vi "Load From XML.vi"(8 "error in":errorcluster, 10 "XML file path":path, 11 "state in":T1) -> (0 "error out":errorcluster, 1 "loaded?":bool, 2 "layout keyword":string, 3 "state out":T1)   [LabVIEW 2010, in "NI_SE_Config Front Panel Layout.lvlib"]
uses:
  NI_SE_Config Front Panel Layout.lvlib
  State.ctl
  VI Info.ctl
  VI Panel Layout/VI Panel Layout.lvclass
  VI Panel Layout/VI Panel Layout.lvclass/VI Panel Layout.ctl
  VI Panel Layout/Get Subpanel VIs.vi
  Check File Path.vi
  XML File Path to VI File Path.vi
  File Name to Width_Height.vi
  <vilib>/Utility/libraryn.llb/Check if File or Folder Exists.vi
  NI_SE_Front Panel Layout.lvlib
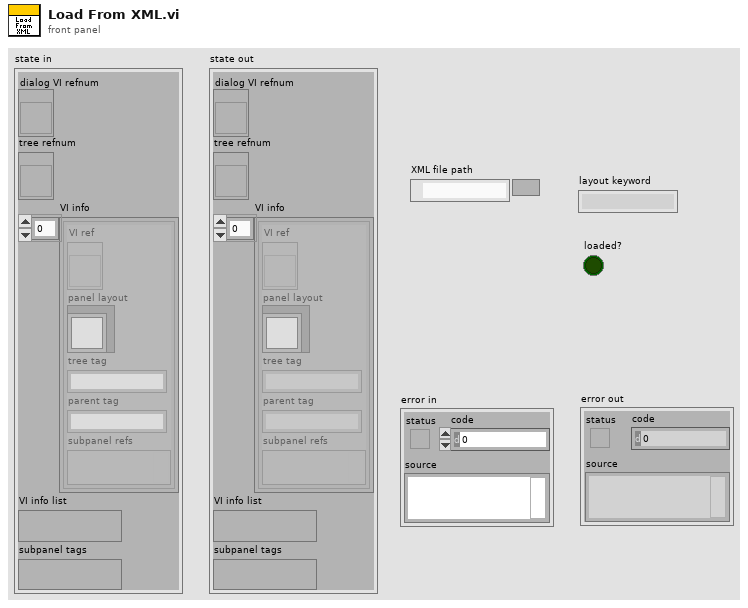
[diagram p1: front panel]
types:
  T1 = typedef "NI_SE_Config Front Panel Layout.lvlib/State.ctl" = cluster{"dialog VI refnum":refnum<vi>, "tree refnum":refnum<vi>, "VI info":T2[], "VI info list":variant, "subpanel tags":variant}
  T2 = typedef "NI_SE_Config Front Panel Layout.lvlib/VI Info.ctl" = cluster{"VI ref":refnum<vi>, "panel layout":refnum<class "VI Panel Layout.lvclass">, "tree tag":string, "parent tag":string, "subpanel refs":variant}
  T3 = typedef "LVBoundsTypeDef.ctl" = cluster{"Width":u32, "Height":u32}
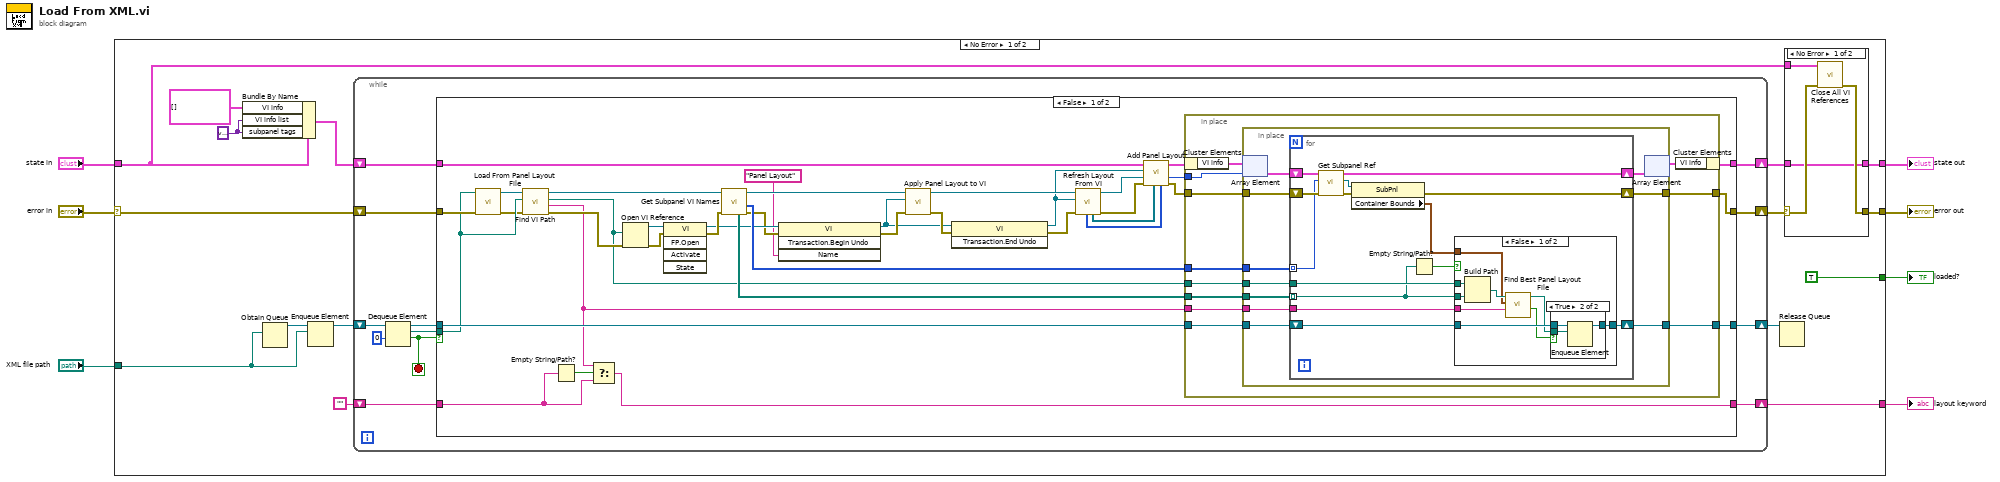
[diagram p0: block diagram]
diagram:
  n1 = case shown="No Error" "error in" {
    selector: "error in" -> [w23 w133]
    tunnel: "state in" -> [w16 w134]
    tunnel: [w8 w134] -> w5
    tunnel: [w14 w133] -> w4
    tunnel: "XML file path" -> [w21 _]
    tunnel: [w12 _] -> w2
    tunnel: [TRUE _] -> w1
    frame No Error {
      w18 = variant ("VI info list")
      n2 = Bundle By Name(cluster=w16, "VI info"=T2[] [], "VI info list"=w18, "subpanel tags"=w18) -> (w15:T1)
      n3 = Obtain Queue(element data type=w21) -> (queue out=w22:refnum<queue>)  [unwired: 4 in, 2 out]
      n4 = Enqueue Element(queue=w22, element=w21) -> (queue out=w20:refnum<queue>)  [unwired: 2 in, 2 out]
      n5 = while {
        shift-right: [w36] -> w19
        shift-left: w20 -> [w40]
        shift-right: [w33] -> w9
        shift-left: w15 -> [w34]
        shift-right: [w32] -> w10
        shift-left: w23 -> [w41]
        shift-right: [w30] -> w12
        shift-left: "" -> [w31]
        stop <- w35 stop-if-true
        n6 = Dequeue Element(queue=w40, timeout in ms (-1)=0) -> (queue out=w37:refnum<queue>, element=w38:path, timed out?=w35:bool)  [unwired: 1 in, 1 out]
        n7 = case shown="False" w35 {
          tunnel: w41 -> [w58 w130]
          tunnel: w38 -> [w54 _]
          tunnel: w37 -> [w78 w132]
          tunnel: [w77 w132] -> w36
          tunnel: w34 -> [w67 w131]
          tunnel: [w65 w131] -> w33
          tunnel: [w61 w130] -> w32
          tunnel: w31 -> [w73 w129]
          tunnel: [w74 w129] -> w30
          frame False {
            n8 = call "Load From Panel Layout File.vi"("error in"=w58, "panel layout file"=w54) -> ("error out"=w53:errorcluster, "panel layout out"=w56:refnum<class "VI Panel Layout.lvclass">)  [unwired: 8 in]
            n9 = call "Find VI Path.vi"("error in (no error)"=w53, "XML path (absolute)"=w54, "VI Panel Layout in"=w56) -> ("error out"=w52:errorcluster, "keyword"=w50:string, "VI path (absolute)"=w51:path, "VI Panel Layout out"=w55:refnum<class "VI Panel Layout.lvclass">)  [unwired: 5 in]
            n10 = Empty String/Path?(string/path=w73) -> (empty?=w75:bool)
            n11 = Select(t=w50, s=w75, f=w73) -> (s? t:f=w74:string)
            n12 = Open VI Reference(vi path=w51, error in (no error)=w52) -> (vi reference=w60:refnum<vi>, error out=w59:errorcluster)  [unwired: 4 in]
            n13 = invoke class="VI" method="FP.Open"(reference=w60, error in=w59) -> (reference out=w49:refnum<vi>, error out=w57:errorcluster)  [unwired: 3 in, 3 out]
            n14 = call "Get Subpanel VI Names.vi"("error in (no error)"=w57, "VI Panel Layout in"=w55) -> ("error out"=w48:errorcluster, "subpanel object UIDs"=w63:i32[], "VI Panel Layout out"=w76:refnum<class "VI Panel Layout.lvclass">, "VI rel paths"=w79:path[])  [unwired: 5 in, 1 out]
            n15 = invoke class="VI" method="Transaction.Begin Undo"(reference=w49, error in=w48, "Name"="Panel Layout") -> (reference out=w43:refnum<vi>, error out=w47:errorcluster)  [unwired: 1 in, 2 out]
            n16 = call "Apply Panel Layout to VI.vi"("error in"=w47, "VI refnum"=w43, "panel layout in"=w76) -> ("error out"=w45:errorcluster, "panel layout out"=w72:refnum<class "VI Panel Layout.lvclass">)  [unwired: 7 in]
            n17 = invoke class="VI" method="Transaction.End Undo"(reference=w43, error in=w45) -> (reference out=w42:refnum<vi>, error out=w44:errorcluster)  [unwired: 1 in, 1 out]
            n18 = call "Refresh Layout From VI.vi"("error in (no error)"=w44, "VI refnum"=w42, "VI Panel Layout in"=w72) -> ("error out"=w70:errorcluster, "VI Panel Layout out"=w71:refnum<class "VI Panel Layout.lvclass">, "subpanel refnums"=w69:refnum<vi>[], "subpanel UIDs"=w68:i32[])  [unwired: 5 in]
            n19 = call "Add Panel Layout.vi"("subpanel UIDs"=w68, "subpanel refnums"=w69, "error in"=w70, "panel layout"=w71, "VI ref"=w42, "state in"=w67) -> ("error out"=w62:errorcluster, "VI info index"=w64:i32, "state out"=w66:T1)  [unwired: 3 in]
            n20 = in-place {
              in-place-border: w79 -> [w90]
              in-place-border: w51 -> [w89]
              in-place-border: w78 -> [w88]
              in-place-border: [w87] -> w77
              in-place-border: w50 -> [w86]
              in-place-border: w64 -> [w83]
              in-place-border: w63 -> [w82]
              in-place-border: w62 -> [w81]
              in-place-border: [w80] -> w61
              n21 = in-place-cluster #1(w66) -> ("VI info"=w85:T2[])
              n22 = in-place {
                in-place-border: w90 -> [w100]
                in-place-border: w89 -> [w99]
                in-place-border: w88 -> [w98]
                in-place-border: [w97] -> w87
                in-place-border: w86 -> [w96]
                in-place-border: w82 -> [w91]
                in-place-border: w81 -> [w93]
                in-place-border: [w92] -> w80
                n23 = in-place-array #2(w85, w83) -> (w95:T2)
                n24 = for {
                  tunnel: w100 -> [w110] mode=indexing
                  tunnel: w99 -> [w114]
                  tunnel: w96 -> [w113]
                  shift-right: [w111] -> w97
                  shift-left: w98 -> [w112]
                  shift-right: [w108] -> w94
                  shift-left: w95 -> [w101]
                  shift-right: [w104] -> w92
                  shift-left: w93 -> [w107]
                  tunnel: w91 -> [w106] mode=indexing
                  n25 = call "Get Subpanel Ref.vi"("error in"=w107, "subpanel UID"=w106, "VI info in"=w101) -> ("error out"=w105:errorcluster, "subpanel ref"=w103:refnum<vi>, "VI info out"=w108:T2)  [unwired: 5 in, 1 out]
                  n26 = property class="SubPnl"(reference=w103, error in=w105) -> (error out=w104:errorcluster, "Container Bounds"=w102:T3)  [unwired: 1 out]
                  n27 = Empty String/Path?(string/path=w110) -> (empty?=w109:bool)
                  n28 = case shown="False" w109 {
                    tunnel: w114 -> [w123 _]
                    tunnel: w113 -> [w121 _]
                    tunnel: w112 -> [w120 w128]
                    tunnel: [w119 w128] -> w111
                    tunnel: w110 -> [w118 _]
                    tunnel: w102 -> [w117 _]
                    frame False {
                      n29 = Build Path(base path=w123, name or relative path=w118) -> (appended path=w122:path)
                      n30 = call "Find Best Panel Layout File.vi"("keyword to match (\"\")"=w121, "desired panel size ([-1,-1])"=w117, "VI path"=w122) -> ("found?"=w115:bool, "panel layout file"=w116:path)  [unwired: 6 in, 1 out]
                      n31 = case shown="True" w115 {
                        tunnel: w120 -> [w124 w127]
                        tunnel: [w124 w126] -> w119
                        tunnel: w116 -> [_ w125]
                        frame False {
                        }
                        frame True {
                          n32 = Enqueue Element(queue=w127, element=w125) -> (queue out=w126:refnum<queue>)  [unwired: 2 in, 2 out]
                        }
                      }
                    }
                    frame True {
                    }
                  }
                }
                n33 = in-place-array #2(w94) -> (w84:T2[])  [unwired: 1 out]
              }
              n34 = in-place-cluster #1("VI info"=w84) -> (w65:T1)
            }
          }
          frame True {
            # "No more files to load."
          }
        }
      }
      n35 = Release Queue(queue=w19) -> ()  [unwired: 2 in, 3 out]
      n36 = case shown="No Error" w10 {
        selector: w10 -> [w25 w29]
        tunnel: w16 -> [w27 w28]
        tunnel: [w26 w29] -> w14
        tunnel: w9 -> [w24 _]
        tunnel: [w24 w28] -> w8
        frame No Error {
          n37 = call "Close All VI References.vi"("error in"=w25, "state in"=w27) -> ("error out"=w26:errorcluster)  [unwired: 9 in]
        }
        frame Error {
        }
      }
    }
    frame Error {
    }
  }
  "state out" <- w5
  "error out" <- w4
  "layout keyword" <- w2
  "loaded?" <- w1
